vi "Dia 1 - strings.vi"() -> ()   [LabVIEW 2014]
panel:
  out "concatenated string":string
  out "error out":errorcluster
  in  "stop":bool
  in  "access (0:read/write)":enum16{"read/write", "read-only", "write-only"}(ring)
  in  "operation (0:open)":T1(ring)
  in  "file path (use dialog)":path
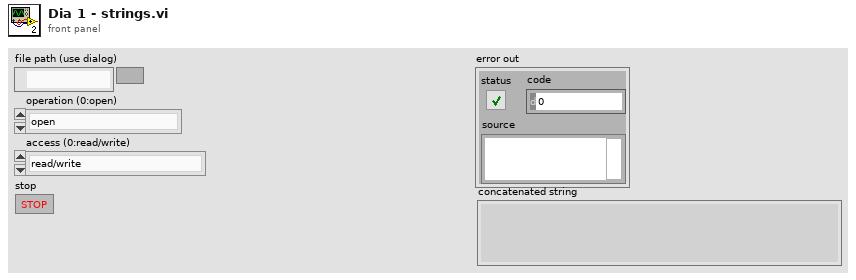
[diagram p1: front panel]
types:
  T1 = enum16{"open", "replace", "create", "open or create", "replace or create", "replace or create with confirmation"}
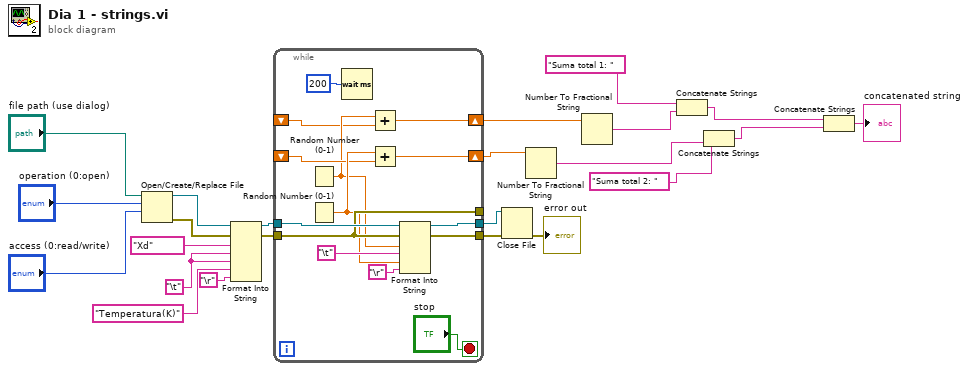
[diagram p0: block diagram]
diagram:
  w12 = "\t"
  n1 = Open/Create/Replace File(file path (use dialog)="file path (use dialog)", operation (0:open)="operation (0:open)", access (0:read/write)="access (0:read/write)") -> (refnum out=w16:refnum<file>, error out=w15:errorcluster)  [unwired: 3 in, 1 out]
  n2 = Format Into String(initial string=w16, error in=w15, "Xd", w12, w12, "Temperatura(K)", "\r") -> (resulting string=w14:refnum<file>, error out=w13:errorcluster)  [unwired: 1 in]
  n3 = while {
    tunnel: w14 -> [w33]
    tunnel: [w30] -> _
    tunnel: [w32] -> w20
    tunnel: [w31] -> w19
    tunnel: w13 -> [w30]
    shift-right: [w28] -> w6
    shift-left: _ -> [w27]
    shift-right: [w25] -> w9
    shift-left: _ -> [w24]
    stop <- "stop" stop-if-true
    n4 = Random Number (0-1)() -> (number: 0 to 1=w26:dbl)
    n5 = Random Number (0-1)() -> (number: 0 to 1=w29:dbl)
    n6 = Wait (ms)(milliseconds to wait=u32 200) -> ()  [unwired: 1 out]
    n7 = Add(x=w26, y=w24) -> (x+y=w25:dbl)
    n8 = Add(x=w29, y=w27) -> (x+y=w28:dbl)
    n9 = Format Into String(initial string=w33, error in=w30, w26, "\t", w29, "\r") -> (resulting string=w32:refnum<file>, error out=w31:errorcluster)  [unwired: 1 in]
  }
  n10 = Close File(refnum=w20, error in=w19) -> (error out=→"error out":errorcluster)  [unwired: 1 out]
  n11 = Number To Fractional String(number=w6) -> (F-format string=w5:string)  [unwired: 3 in]
  n12 = Number To Fractional String(number=w9) -> (F-format string=w8:string)  [unwired: 3 in]
  n13 = Concatenate Strings("Suma total 1: ", w8) -> (w3:string)
  n14 = Concatenate Strings("Suma total 2: ", w5) -> (w2:string)
  n15 = Concatenate Strings(w3, w2) -> (→"concatenated string":string)
